vi "Read_Binary_Wavedump_File.vi"(7 "Trace":i64, 9 "Test":string(combo), 10 "PMT Number":string) -> (0 "End of file":bool, 3 "Trace":i32[](array[numeric]))   [LabVIEW 2018]
panel:
  out "Waveform Graph":i32[](graph)
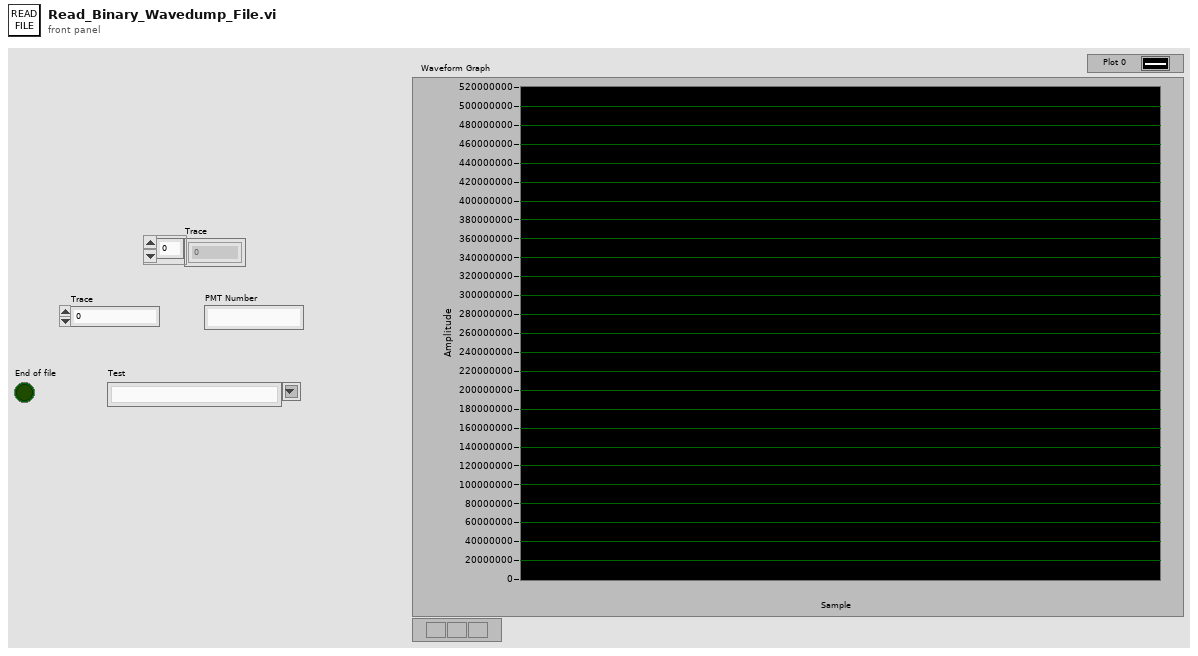
[diagram p1: front panel]
types:
  T1 = enum16{"big-endian, network order", "native, host order", "little-endian"}
  T2 = enum16{"open", "replace", "create", "open or create", "replace or create", "replace or create with confirmation"}
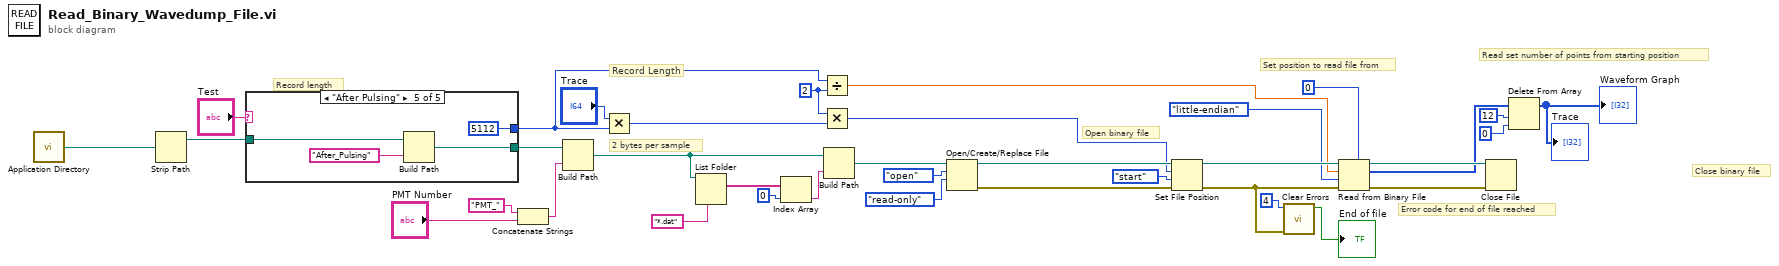
[diagram p0: block diagram]
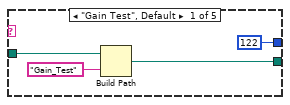
[diagram p2: hidden frame]
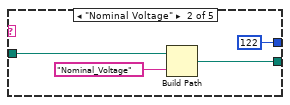
[diagram p3: hidden frame]
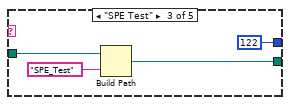
[diagram p4: hidden frame]
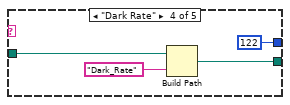
[diagram p5: hidden frame]
diagram:
  w8 = i64 2 ("x")
  # "Record length"
  # "Record Length"
  # "2 bytes per sample"
  # "Error code for end of file reached"
  # "Close binary file"
  # "Read set number of points from starting position"
  # "Set position to read file from"
  # "Open binary file"
  n1 = call <vilib>:"Application Directory.vi"() -> ("Application Directory"=w21:path)
  n2 = Strip Path(path=w21) -> (stripped path=w9:path)  [unwired: 1 out]
  n3 = case shown="\"After Pulsing\"" "Test" {
    tunnel: [w39 w42 w46 w51 w55] -> w10
    tunnel: w9 -> [w38 w43 w47 w50 w54]
    tunnel: [122 ("Points to Plot") 122 ("Points to Plot") 122 ("Points to Plot") 122 ("Points to Plot") 5112 ("Points to Plot")] -> w7
    frame "Gain Test", Default {
      n4 = Build Path(base path=w38, name or relative path="Gain_Test") -> (appended path=w39:path)
    }
    frame "Nominal Voltage" {
      n5 = Build Path(base path=w43, name or relative path="Nominal_Voltage") -> (appended path=w42:path)
    }
    frame "SPE Test" {
      n6 = Build Path(base path=w47, name or relative path="SPE_Test") -> (appended path=w46:path)
    }
    frame "Dark Rate" {
      n7 = Build Path(base path=w50, name or relative path="Dark_Rate") -> (appended path=w51:path)
    }
    frame "After Pulsing" {
      n8 = Build Path(base path=w54, name or relative path="After_Pulsing") -> (appended path=w55:path)
    }
  }
  n9 = Concatenate Strings("PMT_" ("name or relative path"), "PMT Number") -> (w19:string)
  n10 = Build Path(base path=w10, name or relative path=w19) -> (appended path=w14:path)
  n11 = Multiply(x="Trace", y=w7) -> (x*y=w5:i64)
  n12 = List Folder(path=w14, pattern="*.dat") -> (filenames=w16:string[])  [unwired: 2 in, 3 out]
  n13 = Index Array(array=w16, index=0) -> (element=w13:string)
  n14 = Divide(x=w7, y=w8) -> (x/y=w22:dbl)
  n15 = Multiply(x=w8, y=w5) -> (x*y=w23:i64)
  n16 = Build Path(base path=w14, name or relative path=w13) -> (appended path=w12:path)
  n17 = Open/Create/Replace File(file path (use dialog)=w12, operation (0:open)=T2."open", access (0:read/write)=enum16{"read/write", "read-only", "write-only"}."read-only") -> (refnum out=w30:refnum<file>, error out=w34:errorcluster)  [unwired: 3 in, 1 out]
  n18 = Set File Position(offset (in bytes) (0)=w23, refnum=w30, from (0:start)=enum16{"start", "end", "current"}."start", error in=w34) -> (refnum out=w29:refnum<file>, error out=w35:errorcluster)
  n19 = call <vilib>:"Clear Errors.vi"("error in (no error)"=w35, "specific error code to clear (0: all)"=4) -> ("specific error cleared?"=→"End of file":bool)  [unwired: 4 in, 1 out]
  n20 = Read from Binary File(5:0, 8:w35, 9:T1."little-endian" ("byte order (0:big-endian, network order)"), 10:w22, 11:w29) -> (0:w32:errorcluster, 2:w4:i32[], 3:w28:refnum<file>)  [unwired: 1 in, 1 out]
  n21 = Close File(refnum=w28, error in=w32) -> ()  [unwired: 2 out]
  n22 = Delete From Array(array=w4, length=12, index=0) -> (array with subset deleted=→"Waveform Graph" →"Trace":i32[])  [unwired: 1 out]
